vi "Read Refs.vi"(10 "Refs":refnum<class "Refs.lvclass">) -> (0 "Error out":errorcluster, 2 "Refs":T1)   [LabVIEW 2025, in "_Template.lvlib" / "Templates.lvlib" / "TEMPLATE Actor.lvlib"]
uses:
  TEMPLATE Actor.lvlib
  jettl/jettl/Refs/Refs.lvclass
  Refs.ctl
  TEMPLATE Refs/TEMPLATE Refs.lvclass
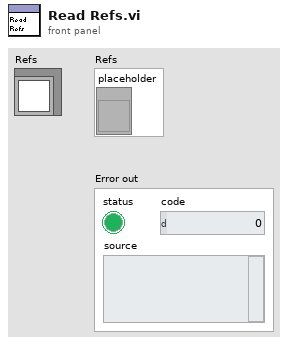
[diagram p1: front panel]
types:
  T1 = typedef "_Template.lvlib/Templates.lvlib/TEMPLATE Actor.lvlib/Refs.ctl" = cluster{"placeholder":refnum<vi>}
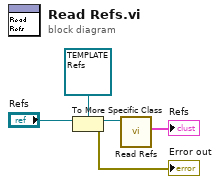
[diagram p0: block diagram]
diagram:
  n1 = To More Specific Class(target class=refnum<class "TEMPLATE Refs.lvclass"> refnum ("_Template.lvlib:Templates.lvlib:TEMPLATE Actor.lvlib:TEMPLATE Refs.lvclass"), reference="Refs") -> (specific class reference=w2:refnum<class "TEMPLATE Refs.lvclass">, error out=→"Error out":errorcluster)  [unwired: 1 in]
  n2 = call "Read Refs.vi"("TEMPLATE Refs in"=w2) -> ("Refs"=→"Refs":T1)  [unwired: 10 in]
